vi "releaseNotifiers.vi"(8 "error in (no error)":errorcluster, 11 "tcpServerBase in":refnum<class "TcpServerBase.lvclass">) -> (0 "error out":errorcluster, 3 "tcpServerBase out":refnum<class "TcpServerBase.lvclass">)   [LabVIEW 2018, in "TcpServerBase.lvclass"]
doc: "Release the notifier references."
uses:
  TcpServerBase.lvclass
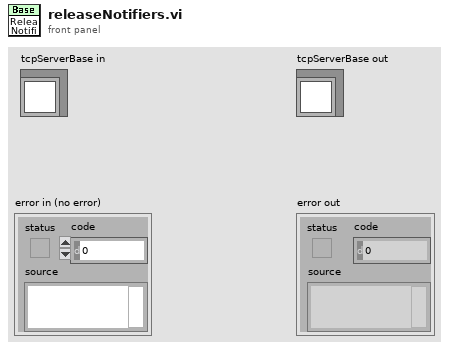
[diagram p1: front panel]
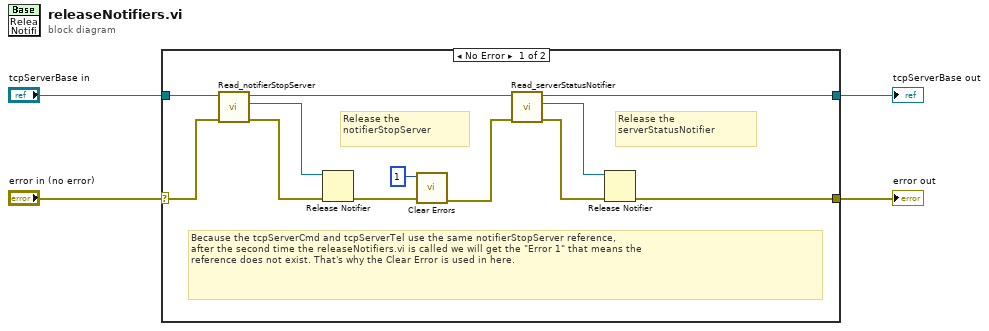
[diagram p0: block diagram]
diagram:
  n1 = case shown="No Error" "error in (no error)" {
    selector: "error in (no error)" -> [w10 w18]
    tunnel: [w5 w18] -> w3
    tunnel: [w16 w17] -> w1
    tunnel: "tcpServerBase in" -> [w11 w17]
    frame No Error {
      # "Because the tcpServerCmd and tcpServerTel use the same notifierStopServer reference,\nafter the second time the releaseNotifiers.vi is called we will get the \"Error 1\" that means the\nreference does not exist. That's why the Clear Error is used in here."
      # "Release the \nserverStatusNotifier"
      # "Release the \nnotifierStopServer"
      n2 = call "Read_notifierStopServer.vi"("error in (no error)"=w10, "TcpServerBase in"=w11) -> ("error out"=w12:errorcluster, "notifierStopServer"=w13:refnum<notifier>, "TcpServerBase out"=w9:refnum<class "TcpServerBase.lvclass">)  [unwired: 7 in]
      n3 = Release Notifier(notifier=w13, error in (no error)=w12) -> (error out=w7:errorcluster)  [unwired: 1 in, 2 out]
      n4 = call <vilib>:"Clear Errors.vi"("error in (no error)"=w7, "specific error code to clear (0: all)"=1) -> ("error out"=w6:errorcluster)  [unwired: 4 in, 1 out]
      n5 = call "Read_serverStatusNotifier.vi"("error in (no error)"=w6, "TcpServerBase in"=w9) -> ("error out"=w15:errorcluster, "serverStatusNotifier"=w14:refnum<notifier>, "TcpServerBase out"=w16:refnum<class "TcpServerBase.lvclass">)  [unwired: 7 in]
      n6 = Release Notifier(notifier=w14, error in (no error)=w15) -> (error out=w5:errorcluster)  [unwired: 1 in, 2 out]
    }
    frame Error {
    }
  }
  "error out" <- w3
  "tcpServerBase out" <- w1
